vi "Power Switch.vi"(0 "P CH":bool, 5 "P CH Used":bool, 7 "Stop":bool, 9 "In1_Shift Register":bool, 11 "In2_Shift Register":bool) -> (10 "Out1_Shift Register":bool, 15 "Out2_Shift Register":bool)   [LabVIEW 2018]
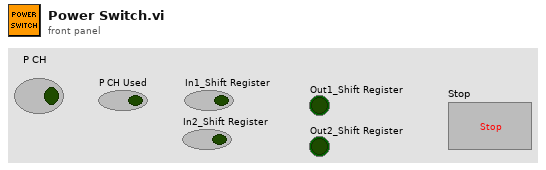
[diagram p1: front panel]
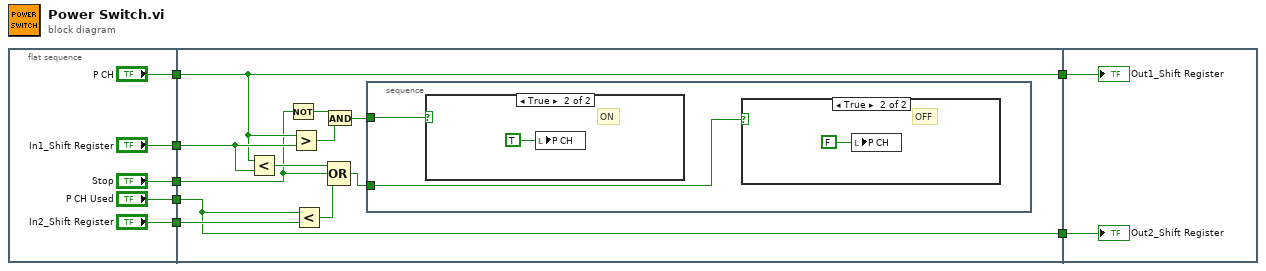
[diagram p0: block diagram]
diagram:
  n1 = flat-sequence {
    tunnel: ["In1_Shift Register"] -> w7
    tunnel: ["P CH Used"] -> w6
    tunnel: ["In2_Shift Register"] -> w5
    tunnel: ["Stop"] -> w4
    tunnel: ["P CH"] -> w3
    tunnel: w7 -> [w17]
    tunnel: w6 -> [w14]
    tunnel: w5 -> [w16]
    tunnel: w4 -> [w13]
    tunnel: w3 -> [w15]
    tunnel: [w15] -> w2
    tunnel: [w14] -> w1
    tunnel: w2 -> [w29]
    tunnel: w1 -> [w28]
    frame #0 {
    }
    frame #1 {
      n2 = Less?(x=w15, y=w17) -> (x < y?=w20:bool)
      n3 = Not(x=w13) -> (.not. x?=w22:bool)
      n4 = Greater?(x=w15, y=w17) -> (0:w23:bool)
      n5 = Less?(x=w14, y=w16) -> (x < y?=w19:bool)
      n6 = And(x=w22, y=w23) -> (x .and. y?=w21:bool)
      n7 = Compound Arithmetic op=OR(w20, w13, w19) -> (w18:bool)
      n8 = stacked-sequence {
        tunnel: w21 -> [w25]
        tunnel: w18 -> [w24]
        frame #0 {
          n9 = case shown="True" w25 {
            frame False {
            }
            frame True {
              # "ON"
              n10 = local write "P CH"(TRUE ("P1 CH0")) -> ()
            }
          }
          n11 = case shown="True" w24 {
            frame False {
            }
            frame True {
              # "OFF"
              n12 = local write "P CH"(FALSE ("P1 CH0")) -> ()
            }
          }
        }
      }
    }
    frame #2 {
      "Out1_Shift Register" <- w29
      "Out2_Shift Register" <- w28
    }
  }
